vi "CPTR Align Math.vi"(6 "sync.meas.oversample factor":u16=1, 7 "sync.cptr.period":u16=1, 9 "sync.cptr.adjust":u16=1, 10 "measurement valid":bool, 11 "measurement":u16) -> (1 "new sync.cptr.adjust":u16, 2 "new sync.cptr.adjust valid":bool, 3 "measurement (in sample clocks)":u16)   [LabVIEW 2012, in "ni579x Synchronization v1 FPGA.lvlib"]
doc: "This VI will generate the new CPTR adjust value that will be fed back into the Gen CPTR VI to create a synchronized CPTR. This VI computes the CPTR based on the measurement for the TDC and also the current CPTR adjust amount."
uses:
  <instrlib>/ni579x/Synchronization/v1/FPGA/ni579x Synchronization v1 FPGA.lvlib
  <vilib>/rvi/FXPMathLib/FxpDiv/subVIs/nifxpmath_Div_SimConfig.ctl
  <vilib>/rvi/FXPMathLib/FxpDiv/simVIs/DllFxpDivTemp_sub.vi
  <vilib>/rvi/FXPMathLib/FxpDiv/XNode/nifxpmath_Div.xnode
  <vilib>/rvi/FXPMathLib/FxpSub/XNode/nifxpmath_Sub.xnode
  <vilib>/rvi/FXPMathLib/FxpAdd/XNode/nifxpmath_Add.xnode
  <vilib>/rvi/FXPMathLib/sim/FxpSim.dll
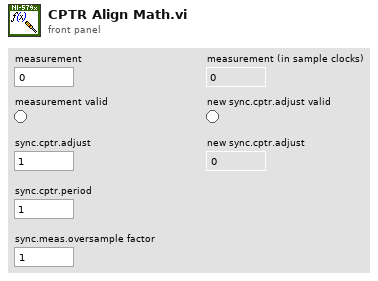
[diagram p1: front panel]
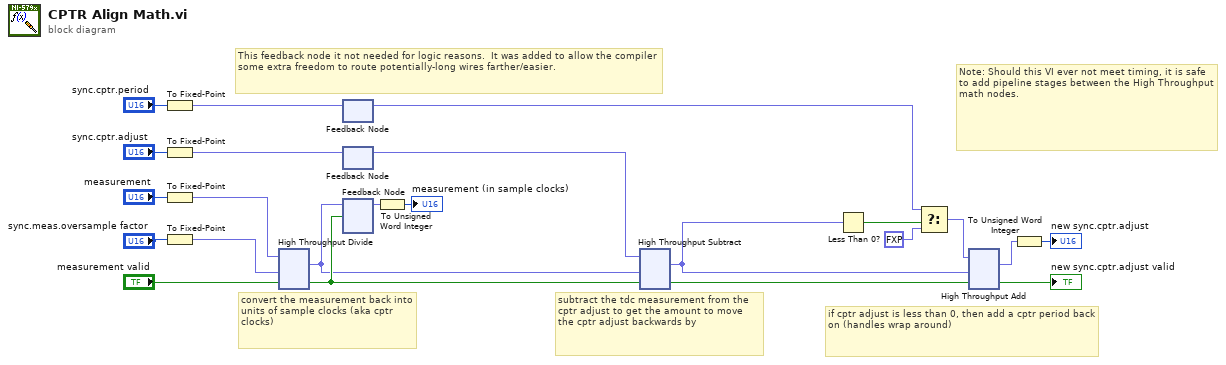
[diagram p0: block diagram]
diagram:
  # "Note: Should this VI ever not meet timing, it is safe to add pipeline stages between the High Throughput math nodes."
  # "This feedback node it not needed for logic reasons.  It was added to allow the compiler some extra freedom to route potentially-long wires farther/easier."
  # "convert the measurement back into units of sample clocks (aka cptr clocks)"
  # "if cptr adjust is less than 0, then add a cptr period back on (handles wrap around)"
  # "subtract the tdc measurement from the cptr adjust to get the amount to move the cptr adjust backwards by"
  n1 = To Fixed-Point(number="sync.cptr.period") -> (fixed-point=w6:fxp<+,16,16>)  [unwired: 1 in]
  n2 = To Fixed-Point(number="sync.cptr.adjust") -> (fixed-point=w4:fxp<+,16,16>)  [unwired: 1 in]
  n3 = To Fixed-Point(number="measurement") -> (fixed-point=w23:fxp<+,16,16>)  [unwired: 1 in]
  n4 = To Fixed-Point(number="sync.meas.oversample factor") -> (fixed-point=w19:fxp<+,16,16>)  [unwired: 1 in]
  n5 = xnode "High Throughput Divide"("x"=w23, "y"=w19, "input valid"="measurement valid") -> ("x/y"=w10:fxp<+,16,16>, "output valid"=w14:bool)  [unwired: 1 in, 1 out]
  n6 = feedback #1() -> (w20:fxp<+,16,16>)  [unwired: 1 in]
  n7 = feedback-in #1(w6) -> ()
  n8 = feedback #2() -> (w3:fxp<+,16,16>)  [unwired: 1 in]
  n9 = feedback-in #2(w4) -> ()
  n10 = feedback #3() -> (w12:fxp<+,16,16>)  [unwired: 1 in]
  n11 = feedback-in #3(w10, w14) -> ()
  n12 = To Unsigned Word Integer(number=w12) -> (unsigned 16bit integer=→"measurement (in sample clocks)":u16)
  n13 = xnode "High Throughput Subtract"("x"=w3, "y"=w10, "input valid"=w14) -> ("x-y"=w13:fxp<+/-,18,18>, "output valid"=w9:bool)  [unwired: 1 in, 1 out]
  n14 = Less Than 0?(x=w13) -> (x < 0?=w22:bool)
  n15 = Select(t=w20, s=w22, f=fxp<+,1,1> 0.0) -> (s? t:f=w5:fxp<+,16,16>)
  n16 = xnode "High Throughput Add"("x"=w5, "y"=w13, "input valid"=w9) -> ("x+y"=w1:fxp<+,16,16>, "output valid"=→"new sync.cptr.adjust valid":bool)  [unwired: 1 in, 1 out]
  n17 = To Unsigned Word Integer(number=w1) -> (unsigned 16bit integer=→"new sync.cptr.adjust":u16)
